vi "Get Inside Terminals.vi"(8 "Error In":errorcluster, 11 "Tunnel in":refnum<vi>) -> (0 "Error Out":errorcluster, 2 "InsideTerms[]":refnum<vi>[](array[refnum]), 3 "Tunnel out":refnum<vi>)   [LabVIEW 2019, in "VI Scripting Tools.lvlib"]
doc: "Use this template to build a VI to use as a subVI."
uses:
  VI Scripting Tools.lvlib
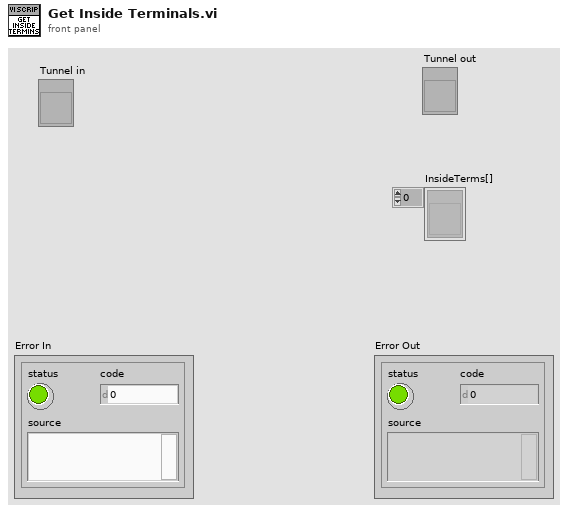
[diagram p1: front panel]
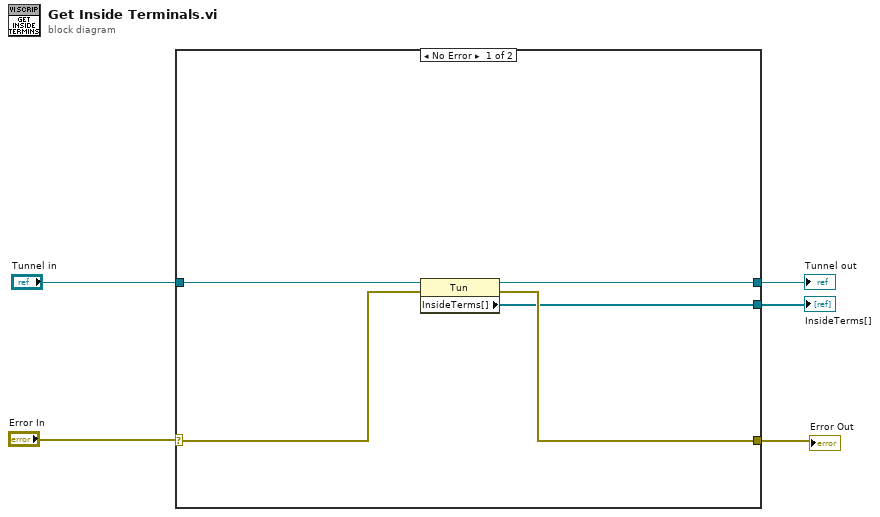
[diagram p0: block diagram]
diagram:
  n1 = case shown="No Error" "Error In" {
    selector: "Error In" -> [w10 w12]
    tunnel: [w8 w12] -> w4
    tunnel: "Tunnel in" -> [w9 w11]
    tunnel: [w7 w11] -> w2
    tunnel: [w6 _] -> w1
    frame No Error {
      n2 = property class="Tun"(reference=w9, error in=w10) -> (reference out=w7:refnum<vi>, error out=w8:errorcluster, "InsideTerms[]"=w6:refnum<vi>[])
    }
    frame Error {
    }
  }
  "Error Out" <- w4
  "Tunnel out" <- w2
  "InsideTerms[]" <- w1
